vi "GEA3 Read ERD (Rev 2 API) Multiple Messages.vi"(0 "GEA2 Reference In":refnum<k24>, 1 "Retry Count":i32=2 min=0 max=255 step=1, 2 "Read Timeout (ms)":u32=500, 5 "GEA Inputs":T4 {"Destination" format="%.0x"; "Source" format="%.0x"}, 7 "Read ERD List":T2[](array[typedef]) {"ERD Number" format="%.0x"}, 11 "Error In":errorcluster, 13 "Verify ERD Response?":bool=TRUE, 14 "Low Level Retry Count":u8=3 min=1 step=1) -> (4 "GEA2 Reference Out":refnum<k24>, 6 "Raw Data Out":string[](array[string]), 8 "ERD Data Out":T1[](array[typedef]) {"ERD Number" format="%.0x"}, 15 "Error Out":errorcluster)   [LabVIEW 2016, in "GEA2_Toolkit.lvlib"]
uses:
  library/GEA2_Toolkit.lvlib
  C:/TechnologyLab/NI-2010/Drivers/GEA3 Toolkit/GEA3 DLL Source/GeaCommunication.dll
  GEA3 DLL Source/GeaCommunication.dll
  type defs/Source_Destination.ctl
  type defs/ERD Read Data In.ctl
  type defs/Data Type.ctl
  type defs/ERD Read Data Out.ctl
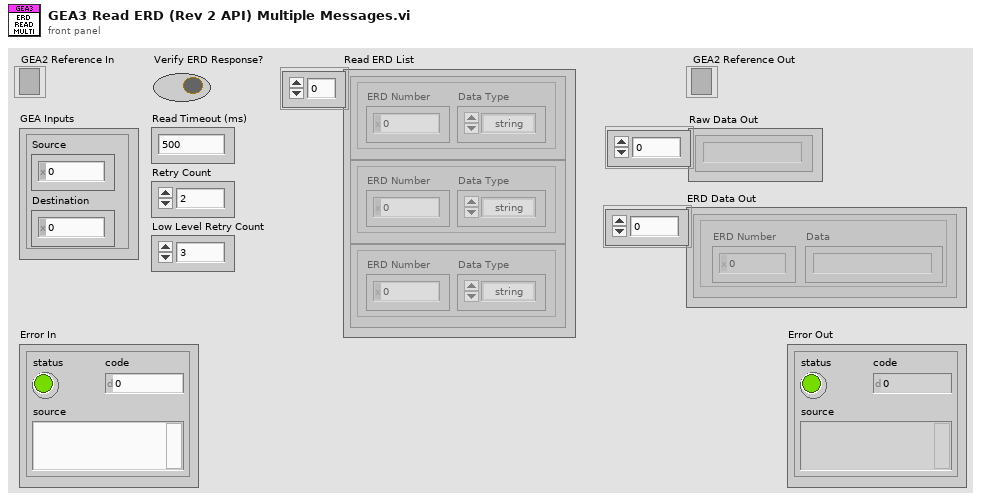
[diagram p1: front panel]
types:
  T1 = typedef "GEA2_Toolkit.lvlib/ERD Read Data Out.ctl" = cluster{"ERD Number":u16, "Data":string}
  T2 = typedef "GEA2_Toolkit.lvlib/ERD Read Data In.ctl" = cluster{"ERD Number":u16, "Data Type":T3}
  T3 = typedef "GEA2_Toolkit.lvlib/Data Type.ctl" = enum16{"string", "boolean", "uint8_t", "uint16_t", "uint32_t", "uint64_t", "int8_t", "int16_t", "int32_t", "int64_t"}
  T4 = typedef "GEA2_Toolkit.lvlib/Source_Destination.ctl" = cluster{"Source":u8, "Destination":u8}
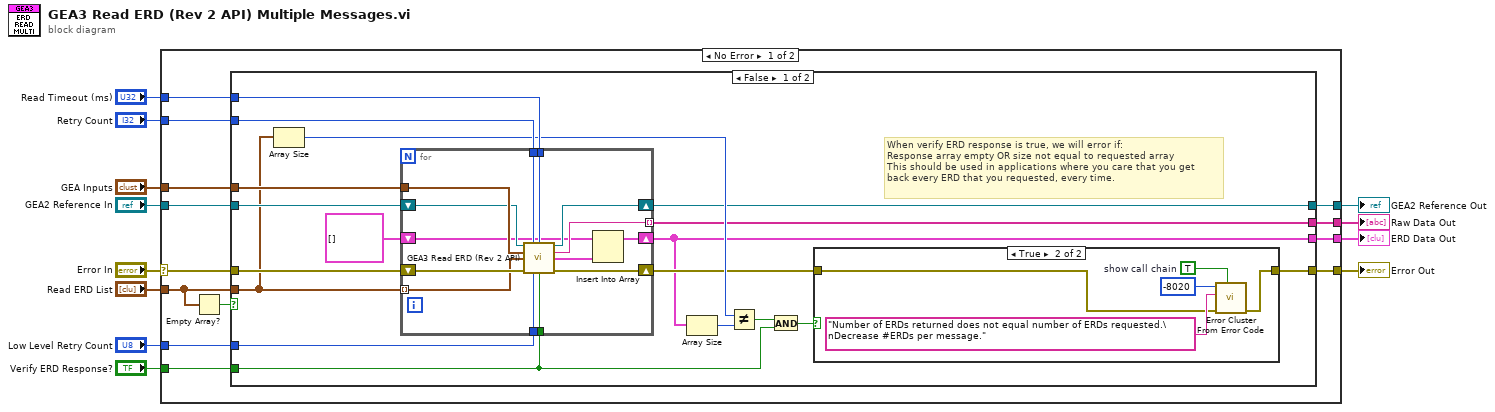
[diagram p0: block diagram]
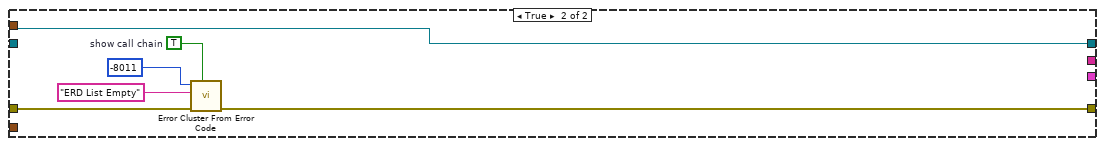
[diagram p3: hidden frame]
diagram:
  n1 = case shown="No Error" "Error In" {
    selector: "Error In" -> [w13 w70]
    tunnel: [w25 w71] -> w12
    tunnel: [w24 w70] -> w11
    tunnel: "Verify ERD Response?" -> [w23 _]
    tunnel: "GEA Inputs" -> [w22 _]
    tunnel: "Read Timeout (ms)" -> [w21 _]
    tunnel: "Retry Count" -> [w20 _]
    tunnel: "GEA2 Reference In" -> [w19 w71]
    tunnel: [w18 _] -> w5
    tunnel: [w17 _] -> w4
    tunnel: "Read ERD List" -> [w16 _]
    tunnel: "Low Level Retry Count" -> [w14 _]
    frame No Error {
      n2 = Empty Array?(array=w16) -> (empty?=w15:bool)
      n3 = case shown="False" w15 {
        tunnel: [w29 w64] -> w25
        tunnel: w13 -> [w43 w66]
        tunnel: [w32 w65] -> w24
        tunnel: w23 -> [w28 _]
        tunnel: w22 -> [w42 _]
        tunnel: w21 -> [w41 _]
        tunnel: w20 -> [w40 _]
        tunnel: w19 -> [w39 w64]
        tunnel: [w30 _] -> w18
        tunnel: [w31 _] -> w17
        tunnel: w16 -> [w36 _]
        tunnel: w14 -> [w37 _]
        frame False {
          # "When verify ERD response is true, we will error if:\nResponse array empty OR size not equal to requested array\nThis should be used in applications where you care that you get\nback every ERD that you requested, every time."
          n4 = Array Size(array=w36) -> (size(s)=w35:i32)
          n5 = for {
            tunnel: w28 -> [w60]
            tunnel: w42 -> [w59]
            tunnel: [w58] -> w30 mode=indexing
            tunnel: w41 -> [w57]
            tunnel: w40 -> [w56]
            shift-right: [w63] -> w29
            shift-left: w39 -> [w55]
            shift-right: [w61] -> w33
            shift-left: w43 -> [w62]
            tunnel: w36 -> [w50] mode=indexing
            shift-right: [w52] -> w31
            shift-left: T1[] [] -> [w54]
            tunnel: w37 -> [w51]
            n6 = call "GEA3 Read ERD (Rev 2 API).vi"("GEA2 Reference In"=w55, "Retry Count"=w56, "Read Timeout (ms)"=w57, "GEA Inputs"=w59, "ERD Read Data In"=w50, "Error In"=w62, "Low Level Tries"=w51, "Verify ERD Response?"=w60) -> ("GEA2 Reference Out"=w63:refnum<k24>, "Raw Data Out"=w58:string, "ERD Read Data Out"=w53:T1, "Error Out"=w61:errorcluster)  [unwired: 4 in]
            n7 = Insert Into Array(array=w54, new element=w53) -> (w52:T1[])  [unwired: 1 in]
          }
          n8 = Array Size(array=w31) -> (size(s)=w34:i32)
          n9 = Not Equal?(x=w35, y=w34) -> (x != y?=w26:bool)
          n10 = And(x=w26, y=w28) -> (x .and. y?=w27:bool)
          n11 = case shown="True" w27 {
            tunnel: w33 -> [w44 w46]
            tunnel: [w44 w45] -> w32
            frame False {
            }
            frame True {
              w49 = TRUE  # show call chain
              n12 = call <vilib>:"Error Cluster From Error Code.vi"("show call chain? (False)"=w49, "error in (no error)"=w46, "error message (\"\")"="Number of ERDs returned does not equal number of ERDs requested.\nDecrease #ERDs per message." ("error message (\"\")"), "error code (0)"=-8020) -> ("error out"=w45:errorcluster)  [unwired: 5 in]
            }
          }
        }
        frame True {
          w67 = TRUE  # show call chain
          n13 = call <vilib>:"Error Cluster From Error Code.vi"("show call chain? (False)"=w67, "error in (no error)"=w66, "error message (\"\")"="ERD List Empty" ("error message (\"\")"), "error code (0)"=-8011) -> ("error out"=w65:errorcluster)  [unwired: 5 in]
        }
      }
    }
    frame Error {
    }
  }
  "GEA2 Reference Out" <- w12
  "Error Out" <- w11
  "Raw Data Out" <- w5
  "ERD Data Out" <- w4
